vi "norm.vi"() -> ()   [LabVIEW 2011]
panel:
  in  "OK Button":bool
  in  "std":dbl
  in  "mean":dbl
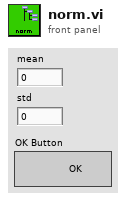
[diagram p1: front panel]
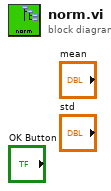
[diagram p0: block diagram]
diagram:
